vi "VdLaser_Create.vi"(0 "reference in":refnum<class "VdLaser.lvclass">, 5 "error in (no error)":errorcluster) -> (14 "reference out":refnum<class "VdLaser.lvclass">, 19 "error out":errorcluster)   [LabVIEW 2010, in "VdLaser.lvclass"]
uses:
  VdLaser.lvclass
  VdLaser.lvclass/VdLaser.ctl
  VdLaser_MyINterface_interface/VdLaser_MyINterface.lvclass
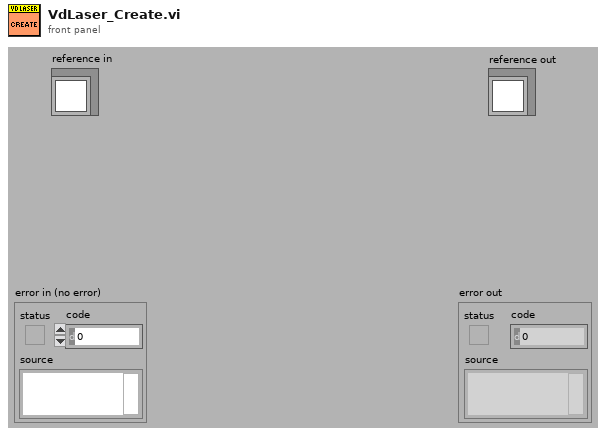
[diagram p1: front panel]
types:
  T1 = typedef "G4BaseTemplate_Simple_6x8x6.lvclass/ObjectAttributes.ctl" = cluster{"Attribute1":dbl}
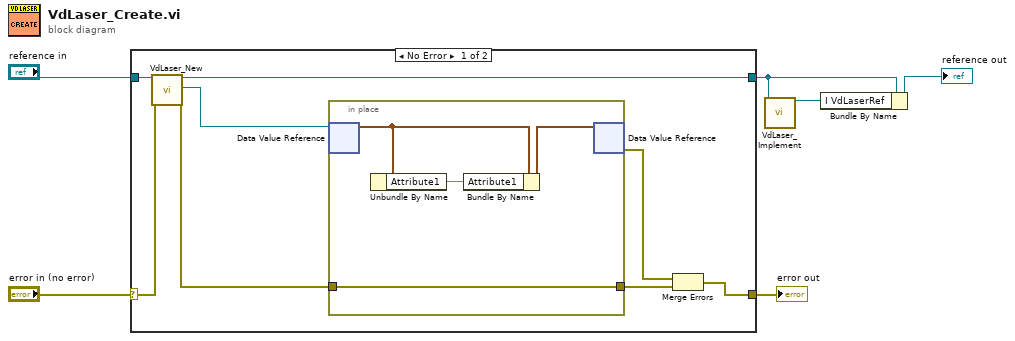
[diagram p0: block diagram]
diagram:
  n1 = case shown="No Error" "error in (no error)" {
    selector: "error in (no error)" -> [w13 w20]
    tunnel: [w10 w20] -> w5
    tunnel: "reference in" -> [w14 w19]
    tunnel: [w12 w19] -> w2
    frame No Error {
      n2 = call "VdLaser_New.vi"("reference in"=w14, "error in (no error)"=w13) -> ("reference out"=w12:refnum<class "VdLaser.lvclass">, "DVRRefOut"=w9:refnum<data-value>, "error out"=w8:errorcluster)  [unwired: 14 in, 1 out]
      n3 = in-place {
        in-place-border: w8 -> [w15]
        in-place-border: [w15] -> w7
        n4 = in-place-dvr #1(w9) -> (w17:T1)  [unwired: 1 out]
        n5 = Unbundle By Name(w17) -> ("Attribute1"=w16:dbl)
        n6 = Bundle By Name(cluster=w17, "Attribute1"=w16) -> (w18:T1)
        n7 = in-place-dvr #1(w18) -> (w11:errorcluster)  [unwired: 1 out]
      }
      n8 = Merge Errors(w11, w7) -> (w10:errorcluster)
    }
    frame Error {
    }
  }
  "error out" <- w5
  n9 = call "VdLaser_Implement.vi"("ClassThatImplements"=w2) -> ("InterfaceHelpClass"=w1:refnum<class "VdLaser_MyINterface.lvclass">)  [unwired: 10 in]
  n10 = Bundle By Name(cluster=w2, "I VdLaserRef"=w1) -> (→"reference out":refnum<class "VdLaser.lvclass">)
